vi "Set Turbo Valve Interlock Configuration.vi"(8 "error in (no error)":errorcluster, 9 "Manual Mode (False)":bool, 10 "Open? (False)":bool, 11 "Turbo in":refnum<class "Turbo.lvclass">) -> (0 "error out":errorcluster, 1 "Interlock Chain":refnum<class "Interlock Chain.lvclass">, 2 "Open? (False) 2":bool, 3 "Turbo out":refnum<class "Turbo.lvclass">)   [LabVIEW 2015, in "cRIO-Carbondioxide.lvlib" / "CO2-Actor.lvlib" / "Turbo.lvclass"]
uses:
  Turbo.lvclass
  Interlocks/Interlock Chain/Interlock Chain.lvclass
  cRIO-CO2/cRIO-CO2.lvclass
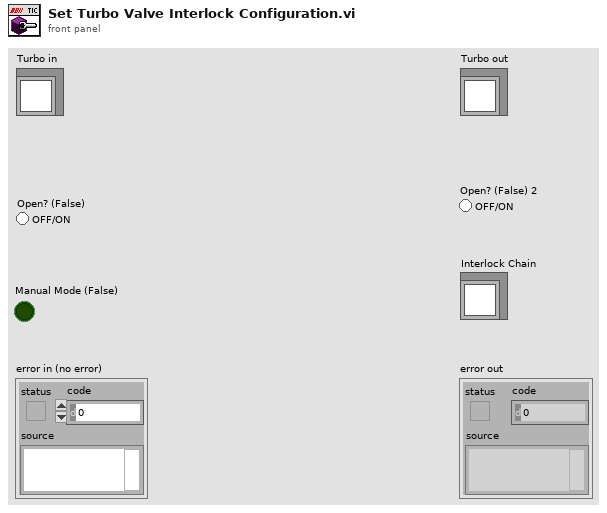
[diagram p1: front panel]
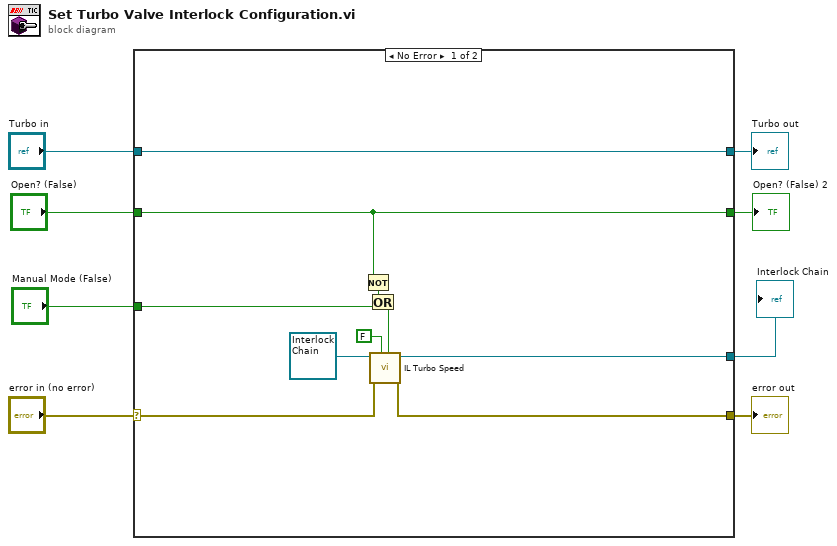
[diagram p0: block diagram]
diagram:
  n1 = case shown="No Error" "error in (no error)" {
    selector: "error in (no error)" -> [w15 w21]
    tunnel: [w14 w21] -> w7
    tunnel: [w17 w20] -> w5
    tunnel: "Turbo in" -> [w17 w20]
    tunnel: "Manual Mode (False)" -> [w18 _]
    tunnel: "Open? (False)" -> [w16 w19]
    tunnel: [w16 w19] -> w2
    tunnel: [w13 _] -> w1
    frame No Error {
      n2 = Not(x=w16) -> (.not. x?=w11:bool)
      n3 = Or(x=w11, y=w18) -> (x .or. y?=w10:bool)
      n4 = call "IL Turbo Speed.vi"("Ignore (F)"=w10, "Stop Self on IL? (T)"=FALSE, "error in (no error)"=w15, "Interlock Chain in"=refnum<class "Interlock Chain.lvclass"> refnum) -> ("error out"=w14:errorcluster, "Interlock Chain out"=w13:refnum<class "Interlock Chain.lvclass">)  [unwired: 5 in, 1 out]
    }
    frame Error {
    }
  }
  "error out" <- w7
  "Turbo out" <- w5
  "Interlock Chain" <- w1
  "Open? (False) 2" <- w2
